vi "Write Start Acquisition.vi"(8 "error in (no error)":errorcluster, 10 "Acquire":bool, 11 "HIJ Vision Camera App in":refnum<class "HIJ Vision Camera App.lvclass">) -> (0 "error out":errorcluster, 3 "HIJ Vision Camera App out":refnum<class "HIJ Vision Camera App.lvclass">)   [LabVIEW 2014, in "HIJ Vision Camera App.lvlib" / "HIJ Vision Camera App.lvclass"]
uses:
  HIJ Vision Camera App.lvclass
  HIJ Vision Camera App.lvclass/HIJ Vision Camera App.ctl
  HIJ Vision Camera App Dialog/HIJ Vision Camera App Dialog/HIJ Vision Camera App Dialog.lvclass/HIJ Vision Camera App Dialog.ctl
  HIJ Vision Camera App Dialog/HIJ Vision Camera App Dialog/Write Acquire.vi
  HIJ Vision Camera App Dialog/HIJ Vision Camera App Dialog/HIJ Vision Camera App Dialog.lvclass
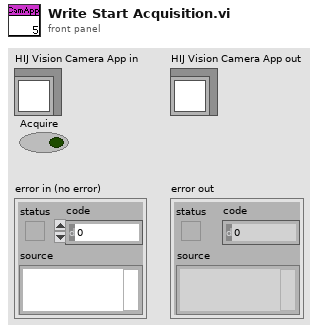
[diagram p1: front panel]
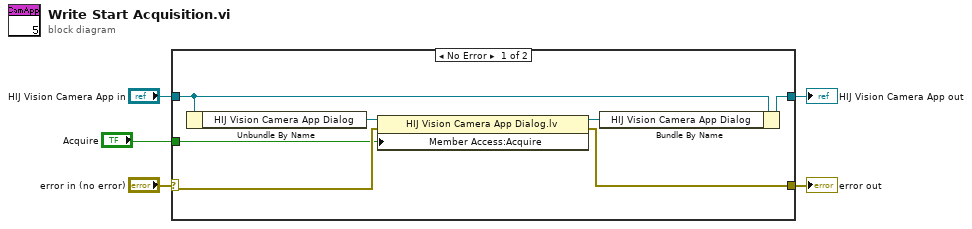
[diagram p0: block diagram]
diagram:
  n1 = case shown="No Error" "error in (no error)" {
    selector: "error in (no error)" -> [w8 w14]
    tunnel: [w7 w14] -> w4
    tunnel: [w10 w13] -> w2
    tunnel: "HIJ Vision Camera App in" -> [w11 w13]
    tunnel: "Acquire" -> [w6 _]
    frame No Error {
      n2 = Unbundle By Name(w11) -> ("HIJ Vision Camera App Dialog"=w12:refnum<class "HIJ Vision Camera App Dialog.lvclass">)
      n3 = property class="HIJ Vision Camera App Dialog.lv"(reference=w12, error in=w8, "Member Access:Acquire"=w6) -> (reference out=w9:refnum<class "HIJ Vision Camera App Dialog.lvclass">, error out=w7:errorcluster)
      n4 = Bundle By Name(cluster=w11, "HIJ Vision Camera App Dialog"=w9) -> (w10:refnum<class "HIJ Vision Camera App.lvclass">)
    }
    frame Error {
    }
  }
  "error out" <- w4
  "HIJ Vision Camera App out" <- w2
